vi "S4GUI.vi"(7 "Tab ObsEng":enum32{"Obs", "CCD modes", "Guider", "Eng"}(tab)) -> ()   [LabVIEW 2018] (continued)
                        # "Polarimetria em aquisição: calcula #PSD"
                        n550 = Unbundle By Name(w1148) -> ("WPROT seq"=w1152:u16)
                        n551 = Number To Boolean Array(number=w1152) -> (Boolean array=w1151:bool[])
                        n552 = for {
                          shift-right: [w1163] -> w1154
                          shift-left: 0 -> [w1161]
                          tunnel: w1151 -> [w1160] mode=indexing
                          # "calcula qtd de 1s"
                          n553 = Increment(x=w1161) -> (x+1=w1162:i32)
                          n554 = Select(t=w1162, s=w1160, f=w1161) -> (s? t:f=w1163:i32)
                        }
                        n555 = property on="#Pol. Seq. Done" class="Slide (strict)"() -> ("Scale.Maximum"=w1153:dbl)  [unwired: 2 in, 2 out]
                        n556 = To Long Integer(number=w1153) -> (32bit integer=w1155:i32)
                        n557 = Subtract(x=w1155, y=w1154) -> (x-y=w1156:i32)
                        n558 = Decrement(x=w1156) -> (x-1=w1158:i32)
                        n559 = Less Than 0?(x=w1158) -> (x < 0?=w1157:bool)
                        n560 = Select(t=0, s=w1157, f=w1158) -> (s? t:f=w1159:i32)
                      }
                    }
                  }
                }
                "#Pol. Seq. Done" <- w1138
                n561 = Number To Decimal String(number=w1138) -> (decimal integer string=w1139:string)  [unwired: 1 in]
                n562 = Concatenate Strings("#Pol. Seq. Done ", w1139) -> (w1137:string)
                n563 = property on="#Pol. Seq. Done" class="Slide (strict)"("Caption.Text"=w1137) -> ()  [unwired: 2 in, 2 out]
              }
              frame #10 {
                # "OVJ 2022-12-12: \nA visibilidade do Tab ObsEng sempre \nacompanha a habilitação do tab4."
                n564 = Unbundle By Name(w1173) -> ("Cluster ExpMode.tab4"=w1167:T12, "Cluster Polarimetry"=w1194:T23, "Cluster Mode Sync"=w1201:T24)
                n565 = case shown="\"Enabled\", Default" w1167 {
                  tunnel: [TRUE ("Tabs Visible?") w1203] -> w1172
                  frame "Enabled", Default {
                  }
                  frame "Disabled and Grayed Out" {
                    n566 = disable-structure shown="Enabled" {
                      disable-tunnel: [TRUE ("Tabs Visible?") FALSE ("Tabs Visible?")] -> w1203
                      frame Disabled {
                        # "DEBUG"
                      }
                      frame Enabled {
                      }
                    }
                  }
                }
                n567 = property on="Tab Acq Type" class="TabCtl (strict)"("DisabledEnum"=w1167) -> (error out=w1171:errorcluster)  [unwired: 2 in, 1 out]
                n568 = Unbundle By Name(w1201) -> ("Start SM Text"=w1200:string, "Star SM"=w1169:T12, "Pause SM"=w1199:T12, "Stop SM"=w1198:T12, "Abort SM"=w1197:T12, "#Cycles"=w1196:T12, "SSM"=w1195:T12, "Set SM"=w1164:T12, "#Index Cycles"=w1170:T12)
                n569 = property on="Observer" class="Str"(error in=w1171, "DisabledEnum"=w1167) -> (error out=w1166:errorcluster)  [unwired: 1 in, 1 out]
                n570 = property on="Tab ObsEng" class="TabCtl (strict)"("Tabs Visible?"=w1172) -> ()  [unwired: 2 in, 2 out]
                n571 = property on="Project ID" class="Str"(error in=w1166, "DisabledEnum"=w1167) -> (error out=w1165:errorcluster)  [unwired: 1 in, 1 out]
                n572 = property on="set keywords" class="Bool"(error in=w1165, "DisabledEnum"=w1164) -> (error out=w1168:errorcluster)  [unwired: 1 in, 1 out]
                n573 = property on="Start SM" class="Bool"("BoolText.Text"=w1200) -> ()  [unwired: 2 in, 2 out]
                n574 = property on="#Cycles Done" class="Slide (strict)"("DisabledEnum"=w1170) -> ()  [unwired: 2 in, 2 out]
                n575 = property on="Start SM" class="Bool"("DisabledEnum"=w1169) -> ()  [unwired: 2 in, 2 out]
                n576 = property on="Stop SM" class="Bool"("DisabledEnum"=w1198) -> ()  [unwired: 2 in, 2 out]
                n577 = property on="Abort SM" class="Bool"("DisabledEnum"=w1197) -> ()  [unwired: 2 in, 2 out]
                n578 = property on="Pause SM" class="Bool"("DisabledEnum"=w1199) -> ()  [unwired: 2 in, 2 out]
                n579 = property on="# Cycles" class="DigNum (strict)"("DisabledEnum"=w1196) -> ()  [unwired: 2 in, 2 out]
                n580 = property on="SSM" class="Ring (strict)"("DisabledEnum"=w1195) -> ()  [unwired: 2 in, 2 out]
                n581 = property on="set Observer" class="Bool"(error in=w1168, "DisabledEnum"=w1164) -> ()  [unwired: 1 in, 2 out]
                n582 = Unbundle By Name(w1194) -> ("Lambda Selector"=w1193:T12, "Calibrator Selector"=w1192:T12, "Set Waveplate"=w1191:T12, "Select Positions"=w1190:T12, "P0"=w1189:T12, "P8"=w1188:T12, "P1"=w1187:T12, "P9"=w1186:T12, "P2"=w1185:T12, "P10"=w1184:T12, "P3"=w1183:T12, "P11"=w1182:T12, "P4"=w1181:T12, "P12"=w1180:T12, "P5"=w1179:T12, "P13"=w1178:T12, "P6"=w1177:T12, "P14"=w1176:T12, "P7"=w1175:T12, "P15"=w1174:T12)
                n583 = property on="P0" class="Bool (strict)"("DisabledEnum"=w1189) -> ()  [unwired: 2 in, 2 out]
                n584 = property on="Lambda Selector" class="Ring (strict)"("DisabledEnum"=w1193) -> ()  [unwired: 2 in, 2 out]
                n585 = property on="Calibrator Selector" class="Ring (strict)"("DisabledEnum"=w1192) -> ()  [unwired: 2 in, 2 out]
                n586 = property on="Set Waveplate" class="Bool"("DisabledEnum"=w1191) -> ()  [unwired: 2 in, 2 out]
                n587 = property on="P1" class="Bool (strict)"("DisabledEnum"=w1187) -> ()  [unwired: 2 in, 2 out]
                n588 = property on="P2" class="Bool (strict)"("DisabledEnum"=w1185) -> ()  [unwired: 2 in, 2 out]
                n589 = property on="Select Positions" class="Ring (strict)"("DisabledEnum"=w1190) -> ()  [unwired: 2 in, 2 out]
                n590 = property on="P3" class="Bool (strict)"("DisabledEnum"=w1183) -> ()  [unwired: 2 in, 2 out]
                n591 = property on="P4" class="Bool (strict)"("DisabledEnum"=w1181) -> ()  [unwired: 2 in, 2 out]
                n592 = property on="P5" class="Bool (strict)"("DisabledEnum"=w1179) -> ()  [unwired: 2 in, 2 out]
                n593 = property on="P6" class="Bool (strict)"("DisabledEnum"=w1177) -> ()  [unwired: 2 in, 2 out]
                n594 = property on="P7" class="Bool (strict)"("DisabledEnum"=w1175) -> ()  [unwired: 2 in, 2 out]
                n595 = property on="P8" class="Bool (strict)"("DisabledEnum"=w1188) -> ()  [unwired: 2 in, 2 out]
                n596 = property on="P9" class="Bool (strict)"("DisabledEnum"=w1186) -> ()  [unwired: 2 in, 2 out]
                n597 = property on="P10" class="Bool (strict)"("DisabledEnum"=w1184) -> ()  [unwired: 2 in, 2 out]
                n598 = property on="P11" class="Bool (strict)"("DisabledEnum"=w1182) -> ()  [unwired: 2 in, 2 out]
                n599 = property on="P12" class="Bool (strict)"("DisabledEnum"=w1180) -> ()  [unwired: 2 in, 2 out]
                n600 = property on="P15" class="Bool (strict)"("DisabledEnum"=w1174) -> ()  [unwired: 2 in, 2 out]
                n601 = property on="P13" class="Bool (strict)"("DisabledEnum"=w1178) -> ()  [unwired: 2 in, 2 out]
                n602 = property on="P14" class="Bool (strict)"("DisabledEnum"=w1176) -> ()  [unwired: 2 in, 2 out]
              }
              frame #11 {
                n603 = Unbundle By Name(w1220) -> ("Cluster Mode CH1"=w1208:T25, "Cluster Mode Sync"=w1207:T24)
                n604 = Unbundle By Name(w1208) -> ("Start ch1 Text"=w1219:string, "#cycles ch1"=w1218:T12, "Start ch1"=w1217:T12, "Pause ch1"=w1216:T12, "Abort ch1"=w1215:T12, "Stop ch1"=w1214:T12, "Exptime ch1"=w1213:T12, "Exp ch1"=w1212:T12, "Set Cooler"=w1206:T12, "Set Temp"=w1211:T12)
                n605 = Unbundle By Name(w1207) -> ("#Index Cycles"=w1210:T12)
                n606 = case shown="Default" w1210 {
                  tunnel: [T12."Enabled" ("#Index Cycles") T12."Disabled and Grayed Out" ("#Index Cycles")] -> w1209
                  frame "Disabled and Grayed Out" {
                  }
                  frame Default {
                  }
                }
                n607 = property on="Start ch1" class="Bool"("BoolText.Text"=w1219) -> ()  [unwired: 2 in, 2 out]
                n608 = property on="Abort ch1" class="Bool"("DisabledEnum"=w1215) -> ()  [unwired: 2 in, 2 out]
                n609 = property on="Set Temp 1" class="Bool"("DisabledEnum"=w1211) -> ()  [unwired: 2 in, 2 out]
                n610 = property on="Stop ch1" class="Bool"("DisabledEnum"=w1214) -> ()  [unwired: 2 in, 2 out]
                n611 = property on="#cycles ch1" class="DigNum (strict)"("DisabledEnum"=w1218) -> ()  [unwired: 2 in, 2 out]
                n612 = property on="cooler ON 1" class="Bool (strict)"("DisabledEnum"=w1206) -> ()  [unwired: 2 in, 2 out]
                n613 = property on="cooler OFF 1" class="Bool (strict)"("DisabledEnum"=w1206) -> ()  [unwired: 2 in, 2 out]
                n614 = property on="Exptime ch1" class="DigNum (strict)"("DisabledEnum"=w1213) -> ()  [unwired: 2 in, 2 out]
                n615 = property on="Start ch1" class="Bool"("DisabledEnum"=w1217) -> ()  [unwired: 2 in, 2 out]
                n616 = property on="Exp ch1" class="DigNum (strict)"("DisabledEnum"=w1212) -> ()  [unwired: 2 in, 2 out]
                n617 = property on="Cycles Done ch1" class="Slide (strict)"("DisabledEnum"=w1209) -> ()  [unwired: 2 in, 2 out]
                n618 = property on="Pause ch1" class="Bool"("DisabledEnum"=w1216) -> ()  [unwired: 2 in, 2 out]
              }
              frame #12 {
                n619 = Unbundle By Name(w1237) -> ("Cluster Mode CH2"=w1236:T26, "Cluster Mode Sync"=w1225:T24)
                n620 = Unbundle By Name(w1225) -> ("#Index Cycles"=w1226:T12)
                n621 = Unbundle By Name(w1236) -> ("Start ch2 Text"=w1235:string, "#cycles ch2"=w1234:T12, "Start ch2"=w1233:T12, "Pause ch2"=w1232:T12, "Stop ch2"=w1231:T12, "Abort ch2"=w1230:T12, "Exptime ch2"=w1229:T12, "Exp ch2"=w1228:T12, "Set Cooler"=w1223:T12, "Set Temp"=w1227:T12)
                n622 = case shown="\"Disabled and Grayed Out\"" w1226 {
                  tunnel: [T12."Enabled" ("#Index Cycles") T12."Disabled and Grayed Out" ("#Index Cycles")] -> w1224
                  frame "Disabled and Grayed Out" {
                  }
                  frame Default {
                  }
                }
                n623 = property on="Start ch2" class="Bool"("BoolText.Text"=w1235) -> ()  [unwired: 2 in, 2 out]
                n624 = property on="Stop ch2" class="Bool"("DisabledEnum"=w1231) -> ()  [unwired: 2 in, 2 out]
                n625 = property on="Abort ch2" class="Bool"("DisabledEnum"=w1230) -> ()  [unwired: 2 in, 2 out]
                n626 = property on="#cycles ch2" class="DigNum (strict)"("DisabledEnum"=w1234) -> ()  [unwired: 2 in, 2 out]
                n627 = property on="Set Temp 2" class="Bool"("DisabledEnum"=w1227) -> ()  [unwired: 2 in, 2 out]
                n628 = property on="Exptime ch2" class="DigNum (strict)"("DisabledEnum"=w1229) -> ()  [unwired: 2 in, 2 out]
                n629 = property on="cooler OFF 2" class="Bool (strict)"("DisabledEnum"=w1223) -> ()  [unwired: 2 in, 2 out]
                n630 = property on="cooler ON 2" class="Bool (strict)"("DisabledEnum"=w1223) -> ()  [unwired: 2 in, 2 out]
                n631 = property on="Start ch2" class="Bool"("DisabledEnum"=w1233) -> ()  [unwired: 2 in, 2 out]
                n632 = property on="Cycles Done ch2" class="Slide (strict)"("DisabledEnum"=w1224) -> ()  [unwired: 2 in, 2 out]
                n633 = property on="Exp ch2" class="DigNum (strict)"("DisabledEnum"=w1228) -> ()  [unwired: 2 in, 2 out]
                n634 = property on="Pause ch2" class="Bool"("DisabledEnum"=w1232) -> ()  [unwired: 2 in, 2 out]
              }
              frame #13 {
                n635 = Unbundle By Name(w1254) -> ("Cluster Mode CH3"=w1253:T27, "Cluster Mode Sync"=w1242:T24)
                n636 = Unbundle By Name(w1242) -> ("#Index Cycles"=w1243:T12)
                n637 = Unbundle By Name(w1253) -> ("Start ch3 Text"=w1252:string, "#cycles ch3"=w1251:T12, "Start ch3"=w1250:T12, "Pause ch3"=w1249:T12, "Stop ch3"=w1248:T12, "Abort ch3"=w1247:T12, "Exptime ch3"=w1246:T12, "Exp ch3"=w1245:T12, "Set Cooler"=w1240:T12, "Set Temp"=w1244:T12)
                n638 = case shown="\"Disabled and Grayed Out\"" w1243 {
                  tunnel: [T12."Enabled" ("#Index Cycles") T12."Disabled and Grayed Out" ("#Index Cycles")] -> w1241
                  frame "Disabled and Grayed Out" {
                  }
                  frame Default {
                  }
                }
                n639 = property on="Start ch3" class="Bool"("BoolText.Text"=w1252) -> ()  [unwired: 2 in, 2 out]
                n640 = property on="Stop ch3" class="Bool"("DisabledEnum"=w1248) -> ()  [unwired: 2 in, 2 out]
                n641 = property on="Abort ch3" class="Bool"("DisabledEnum"=w1247) -> ()  [unwired: 2 in, 2 out]
                n642 = property on="Cycles Done ch3" class="Slide (strict)"("DisabledEnum"=w1241) -> ()  [unwired: 2 in, 2 out]
                n643 = property on="#cycles ch3" class="DigNum (strict)"("DisabledEnum"=w1251) -> ()  [unwired: 2 in, 2 out]
                n644 = property on="cooler OFF 3" class="Bool (strict)"("DisabledEnum"=w1240) -> ()  [unwired: 2 in, 2 out]
                n645 = property on="Set Temp 3" class="Bool"("DisabledEnum"=w1244) -> ()  [unwired: 2 in, 2 out]
                n646 = property on="cooler ON 3" class="Bool (strict)"("DisabledEnum"=w1240) -> ()  [unwired: 2 in, 2 out]
                n647 = property on="Exptime ch3" class="DigNum (strict)"("DisabledEnum"=w1246) -> ()  [unwired: 2 in, 2 out]
                n648 = property on="Start ch3" class="Bool"("DisabledEnum"=w1250) -> ()  [unwired: 2 in, 2 out]
                n649 = property on="Exp ch3" class="DigNum (strict)"("DisabledEnum"=w1245) -> ()  [unwired: 2 in, 2 out]
                n650 = property on="Pause ch3" class="Bool"("DisabledEnum"=w1249) -> ()  [unwired: 2 in, 2 out]
              }
              frame #14 {
                n651 = Unbundle By Name(w1271) -> ("Cluster Mode CH4"=w1270:T28, "Cluster Mode Sync"=w1259:T24)
                n652 = Unbundle By Name(w1259) -> ("#Index Cycles"=w1260:T12)
                n653 = Unbundle By Name(w1270) -> ("Start ch4 Text"=w1269:string, "#cycles ch4"=w1268:T12, "Start ch4"=w1267:T12, "Pause ch4"=w1266:T12, "Stop ch4"=w1265:T12, "Abort ch4"=w1264:T12, "Exptime ch4"=w1263:T12, "Exp ch4"=w1262:T12, "Set Cooler"=w1257:T12, "Set Temp"=w1261:T12)
                n654 = case shown="\"Disabled and Grayed Out\"" w1260 {
                  tunnel: [T12."Enabled" ("#Index Cycles") T12."Disabled and Grayed Out" ("#Index Cycles")] -> w1258
                  frame "Disabled and Grayed Out" {
                  }
                  frame Default {
                  }
                }
                n655 = property on="Start ch4" class="Bool"("BoolText.Text"=w1269) -> ()  [unwired: 2 in, 2 out]
                n656 = property on="Stop ch4" class="Bool"("DisabledEnum"=w1265) -> ()  [unwired: 2 in, 2 out]
                n657 = property on="Abort ch4" class="Bool"("DisabledEnum"=w1264) -> ()  [unwired: 2 in, 2 out]
                n658 = property on="#cycles ch4" class="DigNum (strict)"("DisabledEnum"=w1268) -> ()  [unwired: 2 in, 2 out]
                n659 = property on="Set Temp 4" class="Bool"("DisabledEnum"=w1261) -> ()  [unwired: 2 in, 2 out]
                n660 = property on="cooler ON 4" class="Bool (strict)"("DisabledEnum"=w1257) -> ()  [unwired: 2 in, 2 out]
                n661 = property on="cooler OFF 4" class="Bool (strict)"("DisabledEnum"=w1257) -> ()  [unwired: 2 in, 2 out]
                n662 = property on="Exptime ch4" class="DigNum (strict)"("DisabledEnum"=w1263) -> ()  [unwired: 2 in, 2 out]
                n663 = property on="Cycles Done ch4" class="Slide (strict)"("DisabledEnum"=w1258) -> ()  [unwired: 2 in, 2 out]
                n664 = property on="Start ch4" class="Bool"("DisabledEnum"=w1267) -> ()  [unwired: 2 in, 2 out]
                n665 = property on="Exp ch4" class="DigNum (strict)"("DisabledEnum"=w1262) -> ()  [unwired: 2 in, 2 out]
                n666 = property on="Pause ch4" class="Bool"("DisabledEnum"=w1266) -> ()  [unwired: 2 in, 2 out]
              }
              frame #15 {
                # "Carrega coluna do Channel 1"
                # "Aba:  Eng->Camera"
                n667 = Unbundle By Name(w1338) -> ("ChannelA_CCD"=w1283:T29, "CHA_Checked Params"=w1329:T14, "ChannelA_Status.connection"=w1282:bool)
                n668 = Unbundle By Name(w1329) -> ("ACQUISITION_MODE"=w1307:bool, "TRIGGER_MODE"=w1308:bool, "READ_MODE"=w1309:bool, "PREAMP"=w1317:bool, "READOUT_RATE"=w1318:bool, "VERTICAL_SHIFT_SPEED"=w1319:bool, "EM_MODE"=w1320:bool, "EM_GAIN"=w1310:bool, "SHUTTER_MODE"=w1311:bool, "SHUTTER_TTL"=w1312:bool, "SHUTTER_OPENING_TIME"=w1313:bool, "SHUTTER_CLOSING_TIME"=w1314:bool, "VBIN"=w1315:bool, "HBIN"=w1316:bool, "INITIAL_LINE"=w1321:bool, "INITIAL_COLUMN"=w1326:bool, "FINAL_LINE"=w1328:bool, "FINAL_COLUMN"=w1325:bool, "FRAME_TRANSFER"=w1324:bool, "VERTICAL_CLOCK_VOLTAGE"=w1323:bool, "AD_CHANNEL"=w1322:bool)
                n669 = local read "CH1on"() -> (w1275:bool)
                n670 = Unbundle By Name(w1283) -> ("INITIAL_LINE"=w1305:u16, "INITIAL_COLUMN"=w1304:u16, "FINAL_LINE"=w1303:u16, "FINAL_COLUMN"=w1302:u16, "VBIN"=w1301:u16, "HBIN"=w1300:u16, "PREAMP"=w1299:u8, "EM_GAIN"=w1298:u16, "READOUT_RATE"=w1297:u8, "SHUTTER_OPENNING_TIME"=w1296:u16, "SHUTTER_CLOSING_TIME"=w1295:u16, "VERTICAL_SHIFT_SPEED"=w1294:u8, "READ_MODE"=w1293:u8, "VERTICAL_CLOCK_VOLTAGE"=w1292:u8, "AD_CHANNEL"=w1291:u32, "SHUTTER_MODE"=w1290:u8, "SHUTTER_TTL"=w1289:u8, "TRIGGER_MODE"=w1288:u8, "FRAME_TRANSFER"=w1287:bool, "ACQUISITION_MODE"=w1285:u8, "EM_MODE"=w1284:u8)
                n671 = Equal?(x=w1333, y="none") -> (x = y?=w1330:bool)
                n672 = Equal?(x=w1333, y="default.cfg") -> (x = y?=w1331:bool)
                n673 = Or(x=w1331, y=w1330) -> (x .or. y?=w1332:bool)
                n674 = case shown="True" w1332 {
                  tunnel: [T12."Enabled" ("Disabled") T12."Disabled and Grayed Out" ("Disabled")] -> w1335
                  frame False {
                    # "Se Curr Conf File != default.cfg,\nhabilita botão de Salvar."
                  }
                  frame True {
                    # "Não é permitido salvar em \ncima de default.cfg"
                  }
                }
                n675 = case shown="True" w1282 {
                  tunnel: w1283 -> [_ w1391]
                  tunnel: [w1384 w1390] -> w1281
                  tunnel: [w1384 w1389] -> w1280
                  tunnel: [w1384 w1388] -> w1279
                  tunnel: [w1384 w1387] -> w1278
                  tunnel: [w1384 w1386] -> w1277
                  tunnel: [w1384 w1385] -> w1276
                  frame False {
                    w1384 = "" ("RO1")
                  }
                  frame True {
                    n676 = stacked-sequence "Atualizacao dos indicadores inferiores do CANAL A da tela principal" {
                      tunnel: w1391 -> [w1406 w1409 w1414 w1423 w1426 w1430]
                      tunnel: [w1392 _ _ _ _ _] -> w1390
                      tunnel: [_ w1407 _ _ _ _] -> w1389
                      tunnel: [_ _ w1412 _ _ _] -> w1388
                      tunnel: [_ _ _ w1417 _ _] -> w1387
                      tunnel: [_ _ _ _ w1424 _] -> w1386
                      tunnel: [_ _ _ _ _ w1427] -> w1385
                      frame #0 {
                        # "SubImage"
                        n677 = Unbundle By Name(w1406) -> ("INITIAL_LINE"=w1404:u16, "FINAL_LINE"=w1403:u16, "INITIAL_COLUMN"=w1402:u16, "FINAL_COLUMN"=w1401:u16)
                        n678 = Number To Decimal String(number=w1404) -> (decimal integer string=w1400:string)  [unwired: 1 in]
                        n679 = Number To Decimal String(number=w1403) -> (decimal integer string=w1398:string)  [unwired: 1 in]
                        n680 = Number To Decimal String(number=w1402) -> (decimal integer string=w1396:string)  [unwired: 1 in]
                        n681 = Number To Decimal String(number=w1401) -> (decimal integer string=w1394:string)  [unwired: 1 in]
                        n682 = Concatenate Strings("[", w1400, ":", w1398, ",", w1396, ":", w1394, "]") -> (w1392:string)
                      }
                      frame #1 {
                        # "Em Active"
                        n683 = Unbundle By Name(w1409) -> ("EM_MODE"=w1408:u8)
                        n684 = case shown="0, Default" w1408 {
                          tunnel: ["Electron M." ("EmActive1") "Convent." ("EmActive1")] -> w1407
                          frame 0, Default {
                          }
                          frame 1 {
                          }
                        }
                      }
                      frame #2 {
                        # "Pre Amp"
                        n685 = Unbundle By Name(w1414) -> ("PREAMP"=w1413:u8)
                        n686 = case shown="1" w1413 {
                          tunnel: ["Gain 1" ("EmActive1") "Gain 2" ("EmActive1")] -> w1412
                          frame 0, Default {
                          }
                          frame 1 {
                          }
                        }
                      }
                      frame #3 {
                        # "Binning"
                        n687 = Unbundle By Name(w1423) -> ("VBIN"=w1422:u16, "HBIN"=w1421:u16)
                        n688 = Number To Decimal String(number=w1421) -> (decimal integer string=w1418:string)  [unwired: 1 in]
                        n689 = Number To Decimal String(number=w1422) -> (decimal integer string=w1420:string)  [unwired: 1 in]
                        n690 = Concatenate Strings(w1420, "x", w1418) -> (w1417:string)
                      }
                      frame #4 {
                        # "Gain"
                        n691 = Unbundle By Name(w1426) -> ("EM_GAIN"=w1425:u16)
                        n692 = Number To Decimal String(number=w1425) -> (decimal integer string=w1424:string)  [unwired: 1 in]
                      }
                      frame #5 {
                        # "Readout"
                        n693 = Unbundle By Name(w1430) -> ("EM_MODE"=w1429:u8, "READOUT_RATE"=w1428:u8)
                        n694 = case shown="0, Default" w1429 {
                          tunnel: w1428 -> [w1432 w1438]
                          tunnel: [w1431 w1437] -> w1427
                          frame 0, Default {
                            n695 = case shown="0, Default" w1432 {
                              tunnel: ["30 MHz" ("EmActive1") "20 MHz" ("EmActive1") "10 MHz" ("EmActive1") "1 MHz" ("EmActive1")] -> w1431
                              frame 0, Default {
                              }
                              frame 1 {
                              }
                              frame 2 {
                              }
                              frame 3 {
                              }
                            }
                          }
                          frame 1 {
                            n696 = case shown="1" w1438 {
                              tunnel: ["1 MHz" ("EmActive1") "0.1 MHz" ("EmActive1")] -> w1437
                              frame 0, Default {
                              }
                              frame 1 {
                              }
                            }
                          }
                        }
                      }
                    }
                  }
                }
                n697 = case shown="False" w1275 {
                  tunnel: w1328 -> [_ w1383]
                  tunnel: w1326 -> [_ w1379]
                  tunnel: w1325 -> [_ w1377]
                  tunnel: w1324 -> [_ w1373]
                  tunnel: w1323 -> [_ w1372]
                  tunnel: w1322 -> [_ w1371]
                  tunnel: w1321 -> [_ w1363]
                  tunnel: w1320 -> [_ w1355]
                  tunnel: w1319 -> [_ w1354]
                  tunnel: w1318 -> [_ w1353]
                  tunnel: w1317 -> [_ w1352]
                  tunnel: w1316 -> [_ w1351]
                  tunnel: w1315 -> [_ w1350]
                  tunnel: w1314 -> [_ w1349]
                  tunnel: w1313 -> [_ w1348]
                  tunnel: w1312 -> [_ w1347]
                  tunnel: w1311 -> [_ w1346]
                  tunnel: w1310 -> [_ w1345]
                  tunnel: w1309 -> [_ w1344]
                  tunnel: w1308 -> [_ w1343]
                  tunnel: w1307 -> [_ w1342]
                  tunnel: [T12."Disabled and Grayed Out" ("Disabled") T12."Enabled" ("Disabled")] -> w1274
                  frame False {
                    w1339 = FALSE
                    n698 = property on="Image FInal Column" class="DigNum (strict)"("Blinking"=w1339) -> ()  [unwired: 2 in, 2 out]
                    n699 = property on="Frame Transfer" class="Bool (strict)"("Blinking"=w1339) -> ()  [unwired: 2 in, 2 out]
                    n700 = property on="Vertical Clock Voltage" class="Ring (strict)"("Blinking"=w1339) -> ()  [unwired: 2 in, 2 out]
                    n701 = property on="A/D  Channel" class="DigNum (strict)"("Blinking"=w1339) -> ()  [unwired: 2 in, 2 out]
                    n702 = property on="Image Initial Line" class="DigNum (strict)"("Blinking"=w1339) -> ()  [unwired: 2 in, 2 out]
                    n703 = property on="Image Initial Column" class="DigNum (strict)"("Blinking"=w1339) -> ()  [unwired: 2 in, 2 out]
                    n704 = property on="Image Final Line" class="DigNum (strict)"("Blinking"=w1339) -> ()  [unwired: 2 in, 2 out]
                    n705 = property on="Shutter Openning Time" class="DigNum (strict)"("Blinking"=w1339) -> ()  [unwired: 2 in, 2 out]
                    n706 = property on="Shutter Closing Time" class="DigNum (strict)"("Blinking"=w1339) -> ()  [unwired: 2 in, 2 out]
                    n707 = property on="Vertical Binning" class="DigNum (strict)"("Blinking"=w1339) -> ()  [unwired: 2 in, 2 out]
                    n708 = property on="Horizontal Binning" class="DigNum (strict)"("Blinking"=w1339) -> ()  [unwired: 2 in, 2 out]
                    n709 = property on="CCD EM Gain" class="DigNum (strict)"("Blinking"=w1339) -> ()  [unwired: 2 in, 2 out]
                    n710 = property on="Shutter Mode" class="Ring (strict)"("Blinking"=w1339) -> ()  [unwired: 2 in, 2 out]
                    n711 = property on="Shutter TTL" class="Ring (strict)"("Blinking"=w1339) -> ()  [unwired: 2 in, 2 out]
                    n712 = property on="Acquisition Mode" class="Ring (strict)"("Blinking"=w1339) -> ()  [unwired: 2 in, 2 out]
                    n713 = property on="Readout Rate" class="Ring (strict)"("Blinking"=w1339) -> ()  [unwired: 2 in, 2 out]
                    n714 = property on="Vertical Shift Speed" class="Ring (strict)"("Blinking"=w1339) -> ()  [unwired: 2 in, 2 out]
                    n715 = property on="CCD EM Mode" class="Ring (strict)"("Blinking"=w1339) -> ()  [unwired: 2 in, 2 out]
                    n716 = property on="Trigger Mode" class="Ring (strict)"("Blinking"=w1339) -> ()  [unwired: 2 in, 2 out]
                    n717 = property on="Read Mode" class="Ring (strict)"("Blinking"=w1339) -> ()  [unwired: 2 in, 2 out]
                    n718 = property on="Pre-amplification Gain" class="Ring (strict)"("Blinking"=w1339) -> ()  [unwired: 2 in, 2 out]
                  }
                  frame True {
                    n719 = Not(x=w1377) -> (.not. x?=w1378:bool)
                    n720 = Not(x=w1373) -> (.not. x?=w1375:bool)
                    n721 = Not(x=w1372) -> (.not. x?=w1376:bool)
                    n722 = Not(x=w1371) -> (.not. x?=w1374:bool)
                    n723 = Not(x=w1363) -> (.not. x?=w1381:bool)
                    n724 = Not(x=w1379) -> (.not. x?=w1380:bool)
                    n725 = Not(x=w1383) -> (.not. x?=w1382:bool)
                    n726 = property on="Image FInal Column" class="DigNum (strict)"("Blinking"=w1378) -> ()  [unwired: 2 in, 2 out]
                    n727 = property on="Frame Transfer" class="Bool (strict)"("Blinking"=w1375) -> ()  [unwired: 2 in, 2 out]
                    n728 = property on="Vertical Clock Voltage" class="Ring (strict)"("Blinking"=w1376) -> ()  [unwired: 2 in, 2 out]
                    n729 = property on="A/D  Channel" class="DigNum (strict)"("Blinking"=w1374) -> ()  [unwired: 2 in, 2 out]
                    n730 = property on="Image Initial Line" class="DigNum (strict)"("Blinking"=w1381) -> ()  [unwired: 2 in, 2 out]
                    n731 = property on="Image Initial Column" class="DigNum (strict)"("Blinking"=w1380) -> ()  [unwired: 2 in, 2 out]
                    n732 = property on="Image Final Line" class="DigNum (strict)"("Blinking"=w1382) -> ()  [unwired: 2 in, 2 out]
                    n733 = Not(x=w1348) -> (.not. x?=w1367:bool)
                    n734 = Not(x=w1349) -> (.not. x?=w1369:bool)
                    n735 = Not(x=w1350) -> (.not. x?=w1368:bool)
                    n736 = Not(x=w1351) -> (.not. x?=w1370:bool)
                    n737 = Not(x=w1345) -> (.not. x?=w1365:bool)
                    n738 = Not(x=w1346) -> (.not. x?=w1366:bool)
                    n739 = Not(x=w1347) -> (.not. x?=w1364:bool)
                    n740 = property on="Shutter Openning Time" class="DigNum (strict)"("Blinking"=w1367) -> ()  [unwired: 2 in, 2 out]
                    n741 = property on="Shutter Closing Time" class="DigNum (strict)"("Blinking"=w1369) -> ()  [unwired: 2 in, 2 out]
                    n742 = property on="Vertical Binning" class="DigNum (strict)"("Blinking"=w1368) -> ()  [unwired: 2 in, 2 out]
                    n743 = property on="Horizontal Binning" class="DigNum (strict)"("Blinking"=w1370) -> ()  [unwired: 2 in, 2 out]
                    n744 = property on="CCD EM Gain" class="DigNum (strict)"("Blinking"=w1365) -> ()  [unwired: 2 in, 2 out]
                    n745 = property on="Shutter Mode" class="Ring (strict)"("Blinking"=w1366) -> ()  [unwired: 2 in, 2 out]
                    n746 = property on="Shutter TTL" class="Ring (strict)"("Blinking"=w1364) -> ()  [unwired: 2 in, 2 out]
                    n747 = Not(x=w1342) -> (.not. x?=w1356:bool)
                    n748 = Not(x=w1353) -> (.not. x?=w1359:bool)
                    n749 = Not(x=w1354) -> (.not. x?=w1357:bool)
                    n750 = Not(x=w1355) -> (.not. x?=w1358:bool)
                    n751 = Not(x=w1343) -> (.not. x?=w1361:bool)
                    n752 = Not(x=w1344) -> (.not. x?=w1360:bool)
                    n753 = Not(x=w1352) -> (.not. x?=w1362:bool)
                    n754 = property on="Acquisition Mode" class="Ring (strict)"("Blinking"=w1356) -> ()  [unwired: 2 in, 2 out]
                    n755 = property on="Readout Rate" class="Ring (strict)"("Blinking"=w1359) -> ()  [unwired: 2 in, 2 out]
                    n756 = property on="Vertical Shift Speed" class="Ring (strict)"("Blinking"=w1357) -> ()  [unwired: 2 in, 2 out]
                    n757 = property on="CCD EM Mode" class="Ring (strict)"("Blinking"=w1358) -> ()  [unwired: 2 in, 2 out]
                    n758 = property on="Trigger Mode" class="Ring (strict)"("Blinking"=w1361) -> ()  [unwired: 2 in, 2 out]
                    n759 = property on="Read Mode" class="Ring (strict)"("Blinking"=w1360) -> ()  [unwired: 2 in, 2 out]
                    n760 = property on="Pre-amplification Gain" class="Ring (strict)"("Blinking"=w1362) -> ()  [unwired: 2 in, 2 out]
                  }
                }
                n761 = property on="Save Button" class="Bool (strict)"("DisabledEnum"=w1335) -> ()  [unwired: 2 in, 2 out]
                n762 = First Call?() -> (First Call?: T/F=w1306:bool)
                n763 = case shown="True" w1306 {
                  tunnel: w1305 -> [_ w1461]
                  tunnel: w1304 -> [_ w1460]
                  tunnel: w1303 -> [_ w1459]
                  tunnel: w1302 -> [_ w1458]
                  tunnel: w1301 -> [_ w1457]
                  tunnel: w1300 -> [_ w1456]
                  tunnel: w1299 -> [_ w1455]
                  tunnel: w1298 -> [_ w1454]
                  tunnel: w1297 -> [_ w1453]
                  tunnel: w1296 -> [_ w1452]
                  tunnel: w1295 -> [_ w1451]
                  tunnel: w1294 -> [_ w1450]
                  tunnel: w1293 -> [_ w1449]
                  tunnel: w1292 -> [_ w1448]
                  tunnel: w1291 -> [_ w1447]
                  tunnel: w1290 -> [_ w1446]
                  tunnel: w1289 -> [_ w1445]
                  tunnel: w1288 -> [_ w1444]
                  tunnel: w1287 -> [_ w1443]
                  tunnel: w1285 -> [_ w1442]
                  tunnel: w1284 -> [_ w1441]
                  frame False {
                  }
                  frame True {
                    n764 = local read "Input Cluster"() -> (w1465:T8)
                    n765 = Unbundle By Name(w1465) -> ("Parameters"=w1463:T5)
                    n766 = Bundle By Name(cluster=w1463, "Image \nInitial Line"=w1461, "Image\nInitial Column"=w1460, "Image\nFinal Line"=w1459, "Image\nFInal Column"=w1458, "Vertical\nBinning"=w1457, "Horizontal\nBinning"=w1456, "Pre-amplification\nGain"=w1455, "CCD\nEM Gain"=w1454, "Readout\nRate"=w1453, "Shutter\nOpenning Time"=w1452, "Shutter\nClosing Time"=w1451, "Vertical\nShift Speed"=w1450, "Read\nMode"=w1449, "Vertical\nClock Voltage"=w1448, "A/D \nChannel"=w1447, "Shutter\nMode"=w1446, "Shutter\nTTL"=w1445, "Trigger\nMode"=w1444, "Frame\nTransfer"=w1443, "Acquisition\nMode"=w1442, "CCD \nEM Mode"=w1441) -> (w1462:T5)
                    n767 = Bundle By Name(cluster=w1465, "Parameters"=w1462) -> (w1464:T8)
                    n768 = local write "Input Cluster"(w1464) -> ()
                  }
                }
                n769 = local read "Cameras Cluster"() -> (w1337:T7)
                n770 = Bundle By Name(cluster=w1337, "Current Configuration.Image Initial Line"=w1305, "Current Configuration.Image Initial Column"=w1304, "Current Configuration.Image Final Line"=w1303, "Current Configuration.Image FInal Column"=w1302, "Current Configuration.Vertical Binning"=w1301, "Current Configuration.Horizontal Binning"=w1300, "Current Configuration.Pre-amplification Gain"=w1299, "Current Configuration.CCD EM Gain"=w1298, "Current Configuration.Readout Rate"=w1297, "Current Configuration.Shutter Openning Time"=w1296, "Current Configuration.Shutter Closing Time"=w1295, "Current Configuration.Vertical Shift Speed"=w1294, "Current Configuration.Read Mode"=w1293, "Current Configuration.Vertical Clock Voltage"=w1292, "Current Configuration.A/D  Channel"=w1291, "Current Configuration.Shutter Mode"=w1290, "Current Configuration.Shutter TTL"=w1289, "Current Configuration.Trigger Mode"=w1288, "Current Configuration.Frame Transfer"=w1287, "Current Configuration.Acquisition Mode"=w1285, "Current Configuration.CCD EM Mode"=w1284) -> (w1286:T7)
                n771 = local write "RO1"(w1276) -> ()
                n772 = local write "SI1"(w1281) -> ()
                n773 = local write "EA1"(w1280) -> ()
                n774 = local write "PA1"(w1279) -> ()
                n775 = local write "B1"(w1278) -> ()
                n776 = local write "G1"(w1277) -> ()
                n777 = local write "Cameras Cluster"(w1286) -> ()
                n778 = Compound Arithmetic op=AND(w1307, w1308, w1309, w1317, w1318, w1319, w1320, w1310, w1311, w1312, w1313, w1314, w1315, w1316, w1321, w1326, w1328, w1325, w1324, w1323, w1322) -> (→"CCD checked 1":bool)
                n779 = property on="Shutter Openning Time" class="DigNum (strict)"("DisabledEnum"=w1274) -> ()  [unwired: 2 in, 2 out]
                n780 = property on="Shutter Closing Time" class="DigNum (strict)"("DisabledEnum"=w1274) -> ()  [unwired: 2 in, 2 out]
                n781 = property on="Vertical Binning" class="DigNum (strict)"("DisabledEnum"=w1274) -> ()  [unwired: 2 in, 2 out]
                n782 = property on="Horizontal Binning" class="DigNum (strict)"("DisabledEnum"=w1274) -> ()  [unwired: 2 in, 2 out]
                n783 = property on="CCD EM Gain" class="DigNum (strict)"("DisabledEnum"=w1274) -> ()  [unwired: 2 in, 2 out]
                n784 = property on="Shutter Mode" class="Ring (strict)"("DisabledEnum"=w1274) -> ()  [unwired: 2 in, 2 out]
                n785 = property on="Shutter TTL" class="Ring (strict)"("DisabledEnum"=w1274) -> ()  [unwired: 2 in, 2 out]
                n786 = property on="Acquisition Mode" class="Ring (strict)"("DisabledEnum"=w1274) -> ()  [unwired: 2 in, 2 out]
                n787 = property on="Readout Rate" class="Ring (strict)"("DisabledEnum"=w1274) -> ()  [unwired: 2 in, 2 out]
                n788 = property on="Vertical Shift Speed" class="Ring (strict)"("DisabledEnum"=w1274) -> ()  [unwired: 2 in, 2 out]
                n789 = property on="CCD EM Mode" class="Ring (strict)"("DisabledEnum"=w1274) -> ()  [unwired: 2 in, 2 out]
                n790 = property on="Trigger Mode" class="Ring (strict)"("DisabledEnum"=w1274) -> ()  [unwired: 2 in, 2 out]
                n791 = property on="Read Mode" class="Ring (strict)"("DisabledEnum"=w1274) -> ()  [unwired: 2 in, 2 out]
                n792 = property on="Pre-amplification Gain" class="Ring (strict)"("DisabledEnum"=w1274) -> ()  [unwired: 2 in, 2 out]
                n793 = property on="Image FInal Column" class="DigNum (strict)"("DisabledEnum"=w1274) -> ()  [unwired: 2 in, 2 out]
                n794 = property on="Frame Transfer" class="Bool (strict)"("DisabledEnum"=w1274) -> ()  [unwired: 2 in, 2 out]
                n795 = property on="Vertical Clock Voltage" class="Ring (strict)"("DisabledEnum"=w1274) -> ()  [unwired: 2 in, 2 out]
                n796 = property on="A/D  Channel" class="DigNum (strict)"("DisabledEnum"=w1274) -> ()  [unwired: 2 in, 2 out]
                n797 = property on="Image Initial Line" class="DigNum (strict)"("DisabledEnum"=w1274) -> ()  [unwired: 2 in, 2 out]
                n798 = property on="Image Initial Column" class="DigNum (strict)"("DisabledEnum"=w1274) -> ()  [unwired: 2 in, 2 out]
                n799 = property on="Image Final Line" class="DigNum (strict)"("DisabledEnum"=w1274) -> ()  [unwired: 2 in, 2 out]
                "Current Configuration File:" <- w1333
              }
              frame #16 {
                # "Carrega coluna do Channel 2"
                # "Aba:  Eng->Camera"
                n800 = Unbundle By Name(w1524) -> ("ChannelB_CCD"=w1480:T29, "CHB_Checked Params"=w1481:T14, "ChannelB_Status.connection"=w1479:bool)
                n801 = Unbundle By Name(w1481) -> ("ACQUISITION_MODE"=w1497:bool, "TRIGGER_MODE"=w1496:bool, "READ_MODE"=w1495:bool, "PREAMP"=w1494:bool, "READOUT_RATE"=w1470:bool, "VERTICAL_SHIFT_SPEED"=w1469:bool, "EM_MODE"=w1493:bool, "EM_GAIN"=w1504:bool, "SHUTTER_MODE"=w1503:bool, "SHUTTER_TTL"=w1502:bool, "SHUTTER_OPENING_TIME"=w1501:bool, "SHUTTER_CLOSING_TIME"=w1500:bool, "VBIN"=w1499:bool, "HBIN"=w1498:bool, "INITIAL_LINE"=w1511:bool, "INITIAL_COLUMN"=w1510:bool, "FINAL_LINE"=w1509:bool, "FINAL_COLUMN"=w1508:bool, "FRAME_TRANSFER"=w1507:bool, "VERTICAL_CLOCK_VOLTAGE"=w1506:bool, "AD_CHANNEL"=w1505:bool)
                n802 = case shown="True" w1479 {
                  tunnel: w1480 -> [_ w1581]
                  tunnel: [w1574 w1580] -> w1478
                  tunnel: [w1574 w1579] -> w1477
                  tunnel: [w1574 w1578] -> w1476
                  tunnel: [w1574 w1577] -> w1475
                  tunnel: [w1574 w1576] -> w1474
                  tunnel: [w1574 w1575] -> w1473
                  frame False {
                    w1574 = "" ("EmActive1")
                  }
                  frame True {
                    n803 = stacked-sequence "Atualizacao dos indicadores inferiores do CANAL B da tela principal" {
                      tunnel: w1581 -> [w1596 w1599 w1604 w1613 w1616 w1620]
                      tunnel: [_ w1597 _ _ _ _] -> w1580
                      tunnel: [_ _ w1602 _ _ _] -> w1579
                      tunnel: [_ _ _ w1607 _ _] -> w1578
                      tunnel: [_ _ _ _ w1614 _] -> w1577
                      tunnel: [_ _ _ _ _ w1617] -> w1576
                      tunnel: [w1582 _ _ _ _ _] -> w1575
                      frame #0 {
                        # "SubImage"
                        n804 = Unbundle By Name(w1596) -> ("INITIAL_LINE"=w1594:u16, "FINAL_LINE"=w1593:u16, "INITIAL_COLUMN"=w1592:u16, "FINAL_COLUMN"=w1591:u16)
                        n805 = Number To Decimal String(number=w1594) -> (decimal integer string=w1590:string)  [unwired: 1 in]
                        n806 = Number To Decimal String(number=w1593) -> (decimal integer string=w1588:string)  [unwired: 1 in]
                        n807 = Number To Decimal String(number=w1592) -> (decimal integer string=w1586:string)  [unwired: 1 in]
                        n808 = Number To Decimal String(number=w1591) -> (decimal integer string=w1584:string)  [unwired: 1 in]
                        n809 = Concatenate Strings("[", w1590, ":", w1588, ",", w1586, ":", w1584, "]") -> (w1582:string)
                      }
                      frame #1 {
                        # "Em Active"
                        n810 = Unbundle By Name(w1599) -> ("EM_MODE"=w1598:u8)
                        n811 = case shown="0, Default" w1598 {
                          tunnel: ["Electron M." ("EmActive1") "Convent." ("EmActive1")] -> w1597
                          frame 0, Default {
                          }
                          frame 1 {
                          }
                        }
                      }
                      frame #2 {
                        # "Pre Amp"
                        n812 = Unbundle By Name(w1604) -> ("PREAMP"=w1603:u8)
                        n813 = case shown="1" w1603 {
                          tunnel: ["Gain 1" ("EmActive1") "Gain 2" ("EmActive1")] -> w1602
                          frame 0, Default {
                          }
                          frame 1 {
                          }
                        }
                      }
                      frame #3 {
                        # "Binning"
                        n814 = Unbundle By Name(w1613) -> ("VBIN"=w1612:u16, "HBIN"=w1611:u16)
                        n815 = Number To Decimal String(number=w1611) -> (decimal integer string=w1609:string)  [unwired: 1 in]
                        n816 = Number To Decimal String(number=w1612) -> (decimal integer string=w1610:string)  [unwired: 1 in]
                        n817 = Concatenate Strings(w1610, "x", w1609) -> (w1607:string)
                      }
                      frame #4 {
                        # "Gain"
                        n818 = Unbundle By Name(w1616) -> ("EM_GAIN"=w1615:u16)
                        n819 = Number To Decimal String(number=w1615) -> (decimal integer string=w1614:string)  [unwired: 1 in]
                      }
                      frame #5 {
                        # "Readout"
                        n820 = Unbundle By Name(w1620) -> ("EM_MODE"=w1619:u8, "READOUT_RATE"=w1618:u8)
                        n821 = case shown="0, Default" w1619 {
                          tunnel: w1618 -> [w1622 w1628]
                          tunnel: [w1621 w1627] -> w1617
                          frame 0, Default {
                            n822 = case shown="3" w1622 {
                              tunnel: ["30 MHz" ("EmActive1") "20 MHz" ("EmActive1") "10 MHz" ("EmActive1") "1 MHz" ("EmActive1")] -> w1621
                              frame 0, Default {
                              }
                              frame 1 {
                              }
                              frame 2 {
                              }
                              frame 3 {
                              }
                            }
                          }
                          frame 1 {
                            n823 = case shown="1" w1628 {
                              tunnel: ["1 MHz" ("EmActive1") "0.1 MHz" ("EmActive1")] -> w1627
                              frame 0, Default {
                              }
                              frame 1 {
                              }
                            }
                          }
                        }
                      }
                    }
                  }
                }
                n824 = Unbundle By Name(w1480) -> ("INITIAL_LINE"=w1486:u16, "INITIAL_COLUMN"=w1484:u16, "FINAL_LINE"=w1487:u16, "FINAL_COLUMN"=w1485:u16, "VBIN"=w1490:u16, "HBIN"=w1521:u16, "PREAMP"=w1489:u8, "EM_GAIN"=w1488:u16, "READOUT_RATE"=w1483:u8, "SHUTTER_OPENNING_TIME"=w1520:u16, "SHUTTER_CLOSING_TIME"=w1519:u16, "VERTICAL_SHIFT_SPEED"=w1518:u8, "READ_MODE"=w1517:u8, "VERTICAL_CLOCK_VOLTAGE"=w1516:u8, "AD_CHANNEL"=w1515:u32, "SHUTTER_MODE"=w1512:u8, "SHUTTER_TTL"=w1513:u8, "TRIGGER_MODE"=w1491:u8, "FRAME_TRANSFER"=w1492:bool, "ACQUISITION_MODE"=w1514:u8, "EM_MODE"=w1482:u8)
                n825 = local read "CH2on"() -> (w1472:bool)
                n826 = case shown="False" w1472 {
                  tunnel: w1511 -> [_ w1552]
                  tunnel: w1510 -> [_ w1551]
                  tunnel: w1509 -> [_ w1550]
                  tunnel: w1508 -> [_ w1549]
                  tunnel: w1507 -> [_ w1548]
                  tunnel: w1506 -> [_ w1547]
                  tunnel: w1505 -> [_ w1546]
                  tunnel: w1504 -> [_ w1545]
                  tunnel: w1503 -> [_ w1544]
                  tunnel: w1502 -> [_ w1543]
                  tunnel: w1501 -> [_ w1542]
                  tunnel: w1500 -> [_ w1541]
                  tunnel: w1499 -> [_ w1540]
                  tunnel: w1498 -> [_ w1539]
                  tunnel: w1497 -> [_ w1538]
                  tunnel: w1496 -> [_ w1537]
                  tunnel: w1495 -> [_ w1536]
                  tunnel: w1494 -> [_ w1535]
                  tunnel: w1470 -> [_ w1534]
                  tunnel: w1469 -> [_ w1533]
                  tunnel: w1493 -> [_ w1532]
                  tunnel: [T12."Disabled and Grayed Out" ("Disabled") T12."Enabled" ("Disabled")] -> w1471
                  frame False {
                    w1530 = FALSE ("Blinking")
                    n827 = property on="Image FInal Column 2" class="DigNum (strict)"("Blinking"=w1530) -> ()  [unwired: 2 in, 2 out]
                    n828 = property on="Frame Transfer 2" class="Bool (strict)"("Blinking"=w1530) -> ()  [unwired: 2 in, 2 out]
                    n829 = property on="Vertical Clock Voltage 2" class="Ring (strict)"("Blinking"=w1530) -> ()  [unwired: 2 in, 2 out]
                    n830 = property on="A/D Channel 2" class="DigNum (strict)"("Blinking"=w1530) -> ()  [unwired: 2 in, 2 out]
                    n831 = property on="Image Initial Line 2" class="DigNum (strict)"("Blinking"=w1530) -> ()  [unwired: 2 in, 2 out]
                    n832 = property on="Image Initial Column 2" class="DigNum (strict)"("Blinking"=w1530) -> ()  [unwired: 2 in, 2 out]
                    n833 = property on="Image Final Line 2" class="DigNum (strict)"("Blinking"=w1530) -> ()  [unwired: 2 in, 2 out]
                    n834 = property on="Shutter Openning Time 2" class="DigNum (strict)"("Blinking"=w1530) -> ()  [unwired: 2 in, 2 out]
                    n835 = property on="Shutter Closing Time 2" class="DigNum (strict)"("Blinking"=w1530) -> ()  [unwired: 2 in, 2 out]
                    n836 = property on="Vertical Binning 2" class="DigNum (strict)"("Blinking"=w1530) -> ()  [unwired: 2 in, 2 out]
                    n837 = property on="Horizontal Binning 2" class="DigNum (strict)"("Blinking"=w1530) -> ()  [unwired: 2 in, 2 out]
                    n838 = property on="CCD EM Gain 2" class="DigNum (strict)"("Blinking"=w1530) -> ()  [unwired: 2 in, 2 out]
                    n839 = property on="Shutter Mode 2" class="Ring (strict)"("Blinking"=w1530) -> ()  [unwired: 2 in, 2 out]
                    n840 = property on="Shutter TTL 2" class="Ring (strict)"("Blinking"=w1530) -> ()  [unwired: 2 in, 2 out]
                    n841 = property on="Acquisition Mode 2" class="Ring (strict)"("Blinking"=w1530) -> ()  [unwired: 2 in, 2 out]
                    n842 = property on="Readout Rate 2" class="Ring (strict)"("Blinking"=w1530) -> ()  [unwired: 2 in, 2 out]
                    n843 = property on="Vertical Shift Speed 2" class="Ring (strict)"("Blinking"=w1530) -> ()  [unwired: 2 in, 2 out]
                    n844 = property on="CCD EM Mode 2" class="Ring (strict)"("Blinking"=w1530) -> ()  [unwired: 2 in, 2 out]
                    n845 = property on="Trigger Mode 2" class="Ring (strict)"("Blinking"=w1530) -> ()  [unwired: 2 in, 2 out]
                    n846 = property on="Read Mode 2" class="Ring (strict)"("Blinking"=w1530) -> ()  [unwired: 2 in, 2 out]
                    n847 = property on="Pre-amplification Gain 2" class="Ring (strict)"("Blinking"=w1530) -> ()  [unwired: 2 in, 2 out]
                  }
                  frame True {
                    n848 = Not(x=w1549) -> (.not. x?=w1570:bool)
                    n849 = Not(x=w1548) -> (.not. x?=w1568:bool)
                    n850 = Not(x=w1547) -> (.not. x?=w1569:bool)
                    n851 = Not(x=w1546) -> (.not. x?=w1567:bool)
                    n852 = Not(x=w1552) -> (.not. x?=w1572:bool)
                    n853 = Not(x=w1551) -> (.not. x?=w1571:bool)
                    n854 = Not(x=w1550) -> (.not. x?=w1573:bool)
                    n855 = property on="Image FInal Column 2" class="DigNum (strict)"("Blinking"=w1570) -> ()  [unwired: 2 in, 2 out]
                    n856 = property on="Frame Transfer 2" class="Bool (strict)"("Blinking"=w1568) -> ()  [unwired: 2 in, 2 out]
                    n857 = property on="Vertical Clock Voltage 2" class="Ring (strict)"("Blinking"=w1569) -> ()  [unwired: 2 in, 2 out]
                    n858 = property on="A/D Channel 2" class="DigNum (strict)"("Blinking"=w1567) -> ()  [unwired: 2 in, 2 out]
                    n859 = property on="Image Initial Line 2" class="DigNum (strict)"("Blinking"=w1572) -> ()  [unwired: 2 in, 2 out]
                    n860 = property on="Image Initial Column 2" class="DigNum (strict)"("Blinking"=w1571) -> ()  [unwired: 2 in, 2 out]
                    n861 = property on="Image Final Line 2" class="DigNum (strict)"("Blinking"=w1573) -> ()  [unwired: 2 in, 2 out]
                    n862 = Not(x=w1542) -> (.not. x?=w1563:bool)
                    n863 = Not(x=w1541) -> (.not. x?=w1565:bool)
                    n864 = Not(x=w1540) -> (.not. x?=w1564:bool)
                    n865 = Not(x=w1539) -> (.not. x?=w1566:bool)
                    n866 = Not(x=w1545) -> (.not. x?=w1561:bool)
                    n867 = Not(x=w1544) -> (.not. x?=w1562:bool)
                    n868 = Not(x=w1543) -> (.not. x?=w1560:bool)
                    n869 = property on="Shutter Openning Time 2" class="DigNum (strict)"("Blinking"=w1563) -> ()  [unwired: 2 in, 2 out]
                    n870 = property on="Shutter Closing Time 2" class="DigNum (strict)"("Blinking"=w1565) -> ()  [unwired: 2 in, 2 out]
                    n871 = property on="Vertical Binning 2" class="DigNum (strict)"("Blinking"=w1564) -> ()  [unwired: 2 in, 2 out]
                    n872 = property on="Horizontal Binning 2" class="DigNum (strict)"("Blinking"=w1566) -> ()  [unwired: 2 in, 2 out]
                    n873 = property on="CCD EM Gain 2" class="DigNum (strict)"("Blinking"=w1561) -> ()  [unwired: 2 in, 2 out]
                    n874 = property on="Shutter Mode 2" class="Ring (strict)"("Blinking"=w1562) -> ()  [unwired: 2 in, 2 out]
                    n875 = property on="Shutter TTL 2" class="Ring (strict)"("Blinking"=w1560) -> ()  [unwired: 2 in, 2 out]
                    n876 = Not(x=w1538) -> (.not. x?=w1553:bool)
                    n877 = Not(x=w1534) -> (.not. x?=w1556:bool)
                    n878 = Not(x=w1533) -> (.not. x?=w1554:bool)
                    n879 = Not(x=w1532) -> (.not. x?=w1555:bool)
